vi "align side and front.vi"(8 "error in (no error)":errorcluster, 10 "Target (Volt)":dbl, 11 "Setpoint":dbl) -> (0 "error out":errorcluster)   [LabVIEW 2019]
uses:
  <vilib>/Platform/TimedLoop/XDataNode/timing_clust.ctl
  <vilib>/Platform/TimedLoop/XDataNode/nitl_modes.ctl
  <vilib>/Platform/TimedLoop/XDataNode/wakeup.ctl
  <vilib>/addons/control/pid/pid.llb/PID (DBL).vi
  <vilib>/platform/TimedLoop/XDataNode/XDataNode.xnode
  <vilib>/Platform/TimedLoop/XDataNode/XDNodeRunTimeDep.lvlib
  <vilib>/addons/control/pid/NI_PID_pid.lvlib
panel:
  out "AC estimate (Vrms)":dbl
  out "Waveform Chart 3":dbl(graph)
  out "Waveform Chart 2":dbl(graph)
  out "Waveform Chart":dbl(graph)
  in  "stop":bool
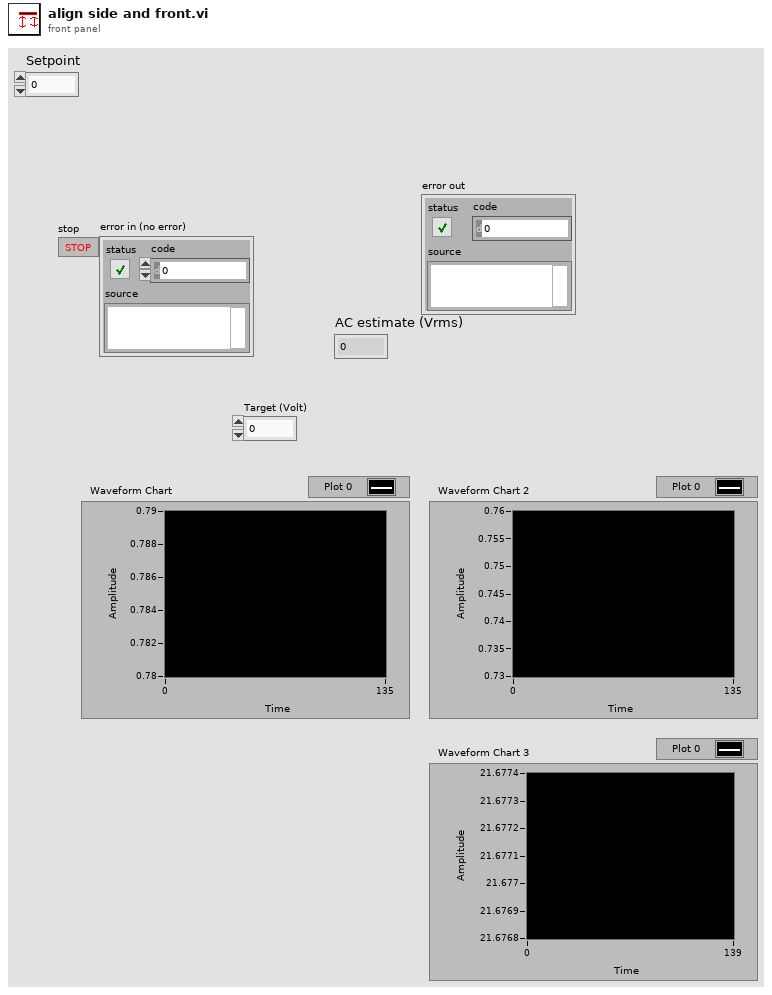
[diagram p1: front panel]
types:
  T1 = typedef "XDNodeRunTimeDep.lvlib/timing_clust.ctl" = cluster{"Expected End [f-1]":u64, "Actual End [f-1]":u64, "Finished Late? [f-1]":bool, "Expected End [i-1]":u64, "Actual End [i-1]":u64, "Finished Late? [i-1]":bool, "Expected Start [i]":u64, "Actual Start [i]":u64, "Expected Start [f]":u64, "Actual Start [f]":u64, "Source Name":string, "Structure Name":string, "Period":i64, "Deadline":i64, "Offset":i64, "Start":i64, "Priority":i32, "Timeout":i32, "Mode":T2, "Wakeup Reason":T3, "Error":errorcluster, "Source Type":string, "Secondary Source Type":string, "Global End Time":u64, "Global Start Time":u64, "Frame Duration":u64, "Iteration Duration":u64, "Assigned CPU":i32, "I/O Scan Engine Mode":u32}
  T2 = typedef "XDNodeRunTimeDep.lvlib/nitl_modes.ctl" = enum32{"No Change", "Process missed periods, maintain original phase", "Discard missed periods, maintain original phase", "Process missed periods, ignore original phase", "Discard missed periods, ignore original phase"}
  T3 = typedef "XDNodeRunTimeDep.lvlib/wakeup.ctl" = enum32{"Normal", "Aborted", "Asynchronous wakeup", "Timing source error", "Timed loop error", "Timeout"}
  T4 = cluster{"proportional gain (Kc)":dbl, "integral time (Ti, min)":dbl, "derivative time (Td, min)":dbl}
  T5 = typedef "IR out.ctl" = cluster{"DC estimate (V) 2":dbl, "DC estimate (V)":dbl, "AC estimate (Vrms)":dbl, "AC estimate (Vrms) 2":dbl}
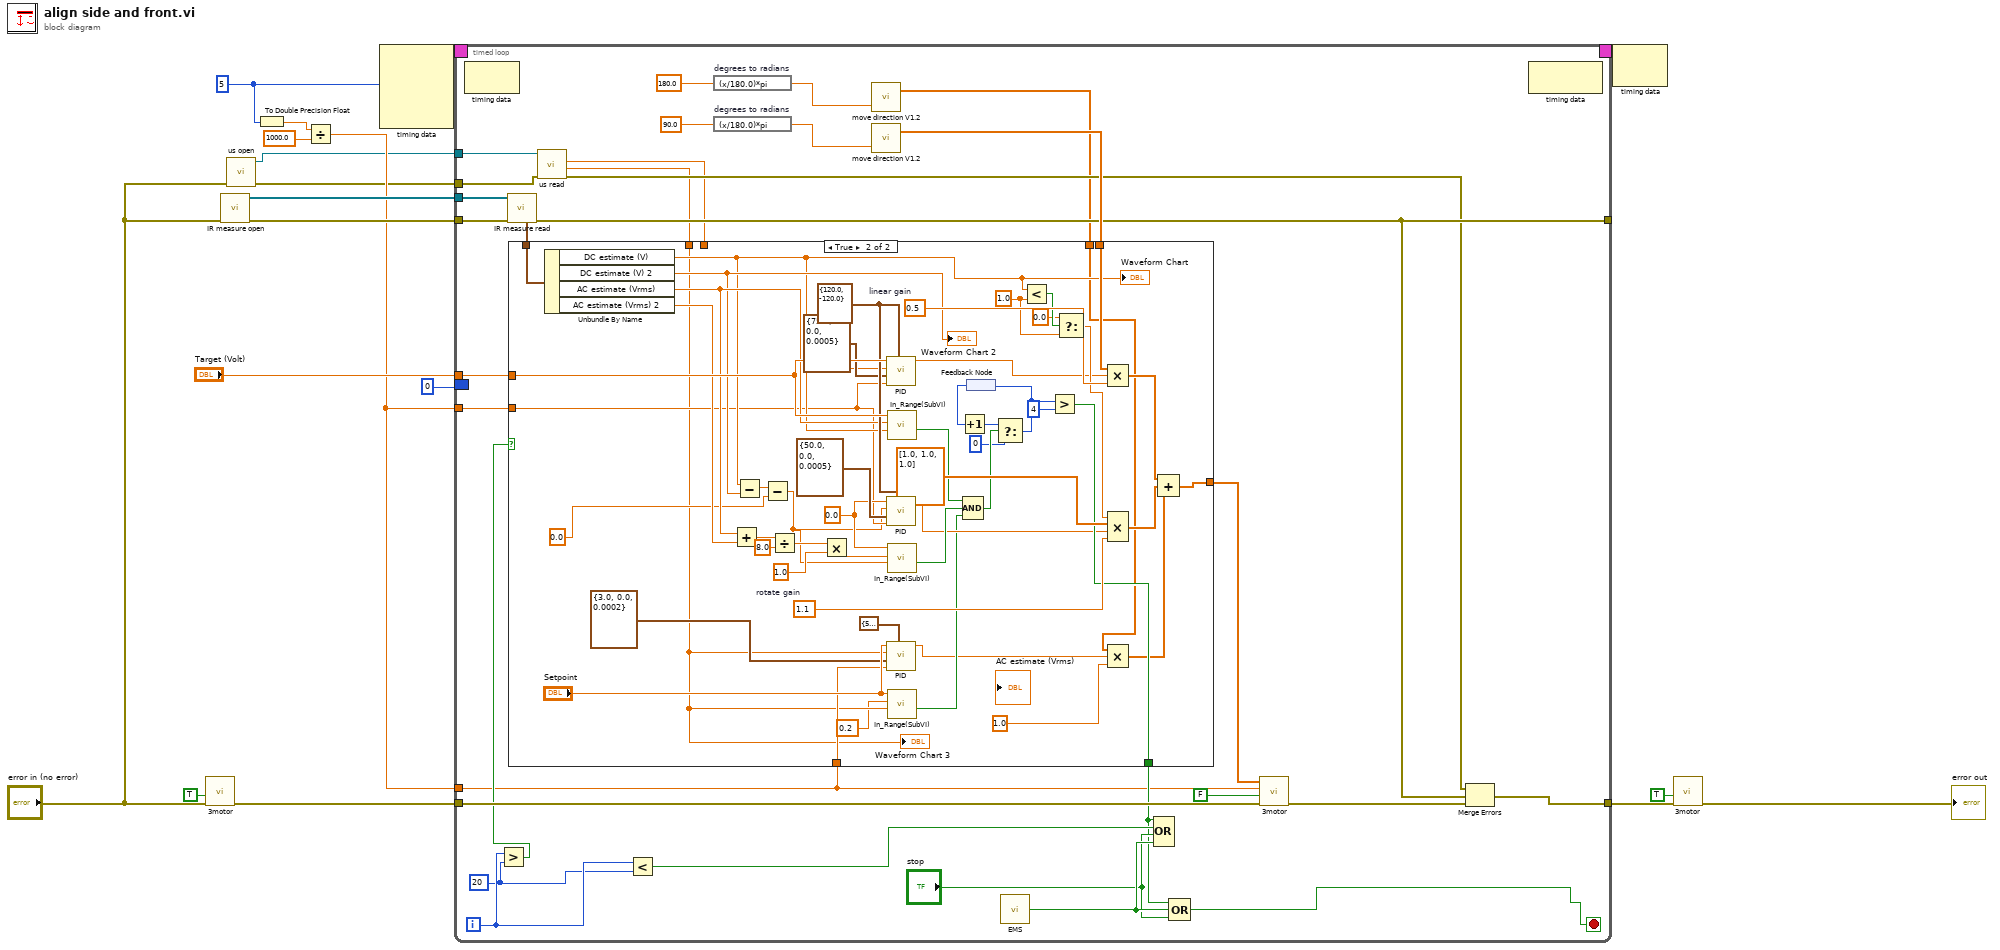
[diagram p0: block diagram]
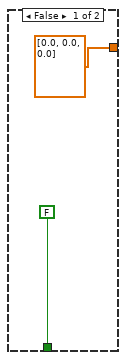
[diagram p2: hidden frame]
diagram:
  w8 = i64 5 ("Period")
  n1 = call "3motor.vi"("error in (no error)"="error in (no error)", "Reset"=TRUE) -> ("error out"=w12:errorcluster)  [unwired: 8 in, 1 out]
  n2 = call "IR measure open.vi"("error in (no error)"="error in (no error)") -> ("error out"=w15:errorcluster, "ref array"=w16:refnum<class "IR sensor.lvclass">[])  [unwired: 9 in]
  n3 = call "us open.vi"("error in"="error in (no error)") -> ("error out"=w2:errorcluster, "output cluster"=w1:refnum<class "US sensor.lvclass">)  [unwired: 9 in]
  n4 = To Double Precision Float(number=w8) -> (double precision float=w7:dbl)
  n5 = Divide(x=w7, y=1000.0) -> (x/y=w4:dbl)
  n6 = node-c288(w8) -> (w18:T1)  [unwired: 3 in]
  n7 = timed-loop {
    timing: w18 -> [_]
    timing-out: [_] -> w17
    tunnel: w16 -> [w49]
    tunnel: [w28] -> _
    tunnel: w15 -> [w48]
    tunnel: "Target (Volt)" -> [w46]
    tunnel: [w29] -> w13
    tunnel: w12 -> [w41]
    tunnel: w4 -> [w22]
    border: 0 -> [_]
    tunnel: w4 -> [w34]
    tunnel: w2 -> [w27]
    tunnel: w1 -> [w26]
    i -> [w38]
    stop <- w33 stop-if-true
    w37 = 20 ("y")
    n8 = node-c288() -> ()  [unwired: 1 in, 1 out]
    n9 = Greater?(x=w38, y=w37) -> (0:w36:bool)
    n10 = call "IR measure read.vi"("error in (no error)"=w48, "ref array"=w49) -> ("error out"=w28:errorcluster, "output cluster"=w47:T5)  [unwired: 7 in, 1 out]
    n11 = call "us read.vi"("Error In"=w27, "my FPGA lib.lvlib:US sensor.lvclass"=w26) -> ("error out"=w25:errorcluster, "DC estimate (V)"=w23:dbl, "AC estimate (Vrms)"=w24:dbl)  [unwired: 5 in, 2 out]
    n12 = Less?(x=w38, y=w37) -> (x < y?=w40:bool)
    n13 = expression code="(x/180.0)*pi" "degrees to radians"(180.0) -> (w20:dbl)
    n14 = expression code="(x/180.0)*pi" "degrees to radians"(90.0) -> (w45:dbl)
    n15 = call "move direction V1.2.vi"("theta"=w20) -> ("out array"=w19:dbl[])  [unwired: 1 in, 1 out]
    n16 = call "move direction V1.2.vi"("theta"=w45) -> ("out array"=w43:dbl[])  [unwired: 1 in, 1 out]
    n17 = case shown="True" w36 {
      tunnel: w47 -> [_ w103]
      tunnel: w46 -> [_ w102]
      tunnel: w43 -> [_ w101]
      tunnel: [FALSE w81] -> w30
      tunnel: [dbl[] [0.0, 0.0, 0.0] w87] -> w39
      tunnel: w34 -> [_ w66]
      tunnel: w24 -> [_ _]
      tunnel: w23 -> [_ w53]
      tunnel: w22 -> [_ w60]
      tunnel: w19 -> [_ w55]
      frame False {
      }
      frame True {
        w75 = 1.0 ("y")
        w100 = 0.5  # linear gain
        w90 = 1.1  # rotate gain
        w97 = 0.0 ("Setpoint")
        w99 = cluster{"output high":dbl, "output low":dbl} {"output high"=120.0, "output low"=-120.0} ("output range")
        n18 = Unbundle By Name(w103) -> ("DC estimate (V)"=w69:dbl, "DC estimate (V) 2"=w82:dbl, "AC estimate (Vrms)"=w96:dbl, "AC estimate (Vrms) 2"=w95:dbl)
        "Waveform Chart" <- w69
        "Waveform Chart 2" <- w82
        n19 = Add(x=w96, y=w95) -> (x+y=w94:dbl)
        n20 = Subtract(x=w69, y=w82) -> (x-y=w64:dbl)
        n21 = Subtract(x=w64, y=0.0 ("align offset")) -> (x-y=w65:dbl)
        n22 = Divide(x=w94, y=8.0) -> (x/y=w92:dbl)
        n23 = Multiply(x=w92, y=1.0) -> (x*y=w73:dbl)
        n24 = call-poly <vilib>:"PID.vi"("output range"=w99, "dt (s)"=w66, "PID gains"=cluster{"Kp":dbl, "Ki":dbl, "Kd":dbl} {"Kp"=75.0, "Ki"=0.0, "Kd"=0.0005} ("PID"), "process variable"=w69, "setpoint"=w102) -> ("output"=w68:dbl)  [unwired: 5 in, 1 out]
        n25 = call-poly <vilib>:"PID.vi"("output range"=w99, "dt (s)"=w66, "PID gains"=cluster{"Kp":dbl, "Ki":dbl, "Kd":dbl} {"Kp"=50.0, "Ki"=0.0, "Kd"=0.0005} ("PID"), "process variable"=w65, "setpoint"=w97) -> ("output"=w67:dbl)  [unwired: 5 in, 1 out]
        n26 = call-poly <vilib>:"PID.vi"("output range"=cluster{"output high":dbl, "output low":dbl} {"output high"=50.0, "output low"=-50.0}, "dt (s)"=w60, "PID gains"=T4 {"proportional gain (Kc)"=3.0, "integral time (Ti, min)"=0.0, "derivative time (Td, min)"=0.0002}, "process variable"=w53, "setpoint"="Setpoint") -> ("output"=w56:dbl)  [unwired: 5 in, 1 out]
        n27 = call "In_Range(SubVI).vi"("Proccess Variable"=w69, "AC estimate (Vrms)"=w96, "Setpoint"=w102) -> ("In Range?"=w80:bool)  [unwired: 7 in, 1 out]
        n28 = call "In_Range(SubVI).vi"("Proccess Variable"=w65, "AC estimate (Vrms)"=w73, "Setpoint"=w97) -> ("In Range?"=w79:bool)  [unwired: 7 in, 1 out]
        n29 = call "In_Range(SubVI).vi"("Proccess Variable"=w53, "AC estimate (Vrms)"=0.2, "Setpoint"="Setpoint") -> ("In Range?"=w57:bool)  [unwired: 7 in, 1 out]
        n30 = Compound Arithmetic op=AND(w80, w79, w57) -> (w78:bool)
        n31 = feedback #1() -> (w85:i32)
        n32 = Increment(x=w85) -> (x+1=w86:i32)
        n33 = Select(t=w86, s=w78, f=0) -> (s? t:f=w84:i32)
        n34 = feedback-in #1(w84) -> ()
        n35 = Less?(x=w69, y=w75) -> (x < y?=w77:bool)
        n36 = Greater?(x=w84, y=4) -> (0:w81:bool)
        n37 = Select(t=0.0, s=w77, f=w75) -> (s? t:f=w74:dbl)
        n38 = Compound Arithmetic op=MULTIPLY(w101, w68, w100) -> (w89:dbl[])
        n39 = Compound Arithmetic op=MULTIPLY(w74, dbl[] [1.0, 1.0, 1.0], w67, w90) -> (w88:dbl[])
        n40 = Compound Arithmetic op=MULTIPLY(w55, w56, 1.0 ("value")) -> (w54:dbl[])
        n41 = Compound Arithmetic op=ADD(w89, w88, w54) -> (w87:dbl[])
        "Waveform Chart 3" <- w53
      }
    }
    n42 = call "EMS.vi"() -> ("A/DIO4 (Pin 19)"=w35:bool)
    n43 = Compound Arithmetic op=OR(w30, w40, "stop", w35) -> ()  [unwired: 1 out]
    n44 = Compound Arithmetic op=OR(w30, w35, "stop") -> (w33:bool)
    n45 = call "3motor.vi"("error in (no error)"=w41, "Reset"=FALSE, "dt(s)"=w22, "Motor speed"=w39) -> ("error out"=w42:errorcluster)  [unwired: 6 in, 1 out]
    n46 = Merge Errors(w25, w28, w42) -> (w29:errorcluster)
    n47 = node-c288() -> ()  [unwired: 1 in, 1 out]
  }
  n48 = node-c288(w17) -> ()  [unwired: 1 out]
  n49 = call "3motor.vi"("error in (no error)"=w13, "Reset"=TRUE) -> ("error out"=→"error out":errorcluster)  [unwired: 8 in, 1 out]
